vi "2.4.vi"() -> ()   [LabVIEW 2020]
panel:
  out "DIVISION":string
  out "PRODUCTO  2":string
  out "RESTA":string
  out "SUMA":string
  in  "Numero B":dbl
  in  "Numero A":dbl
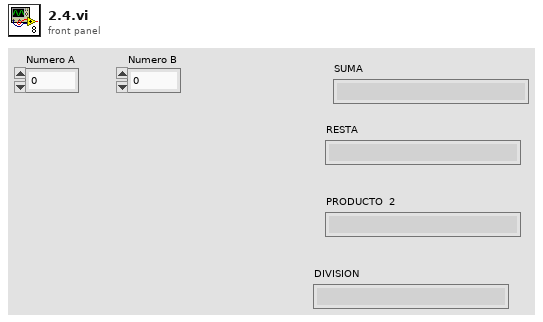
[diagram p1: front panel]
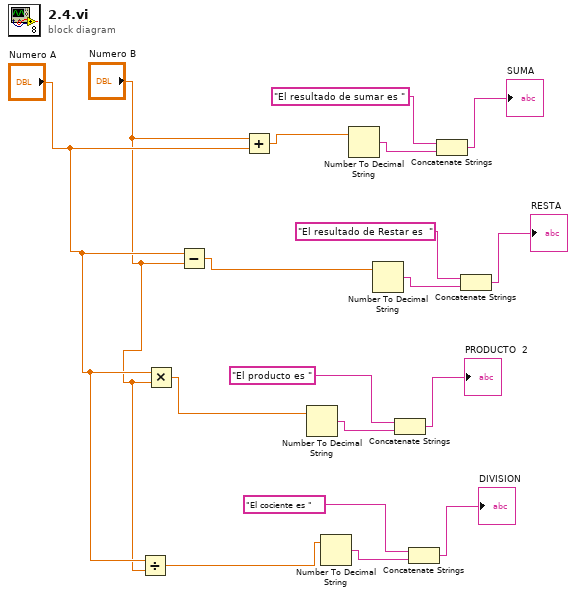
[diagram p0: block diagram]
diagram:
  n1 = Divide(x="Numero A", y="Numero B") -> (x/y=w1:dbl)
  n2 = Multiply(x="Numero A", y="Numero B") -> (x*y=w2:dbl)
  n3 = Subtract(x="Numero A", y="Numero B") -> (x-y=w5:dbl)
  n4 = Add(x="Numero B", y="Numero A") -> (x+y=w18:dbl)
  n5 = Number To Decimal String(number=w2) -> (decimal integer string=w9:string)  [unwired: 1 in]
  n6 = Number To Decimal String(number=w1) -> (decimal integer string=w6:string)  [unwired: 1 in]
  n7 = Number To Decimal String(number=w18) -> (decimal integer string=w15:string)  [unwired: 1 in]
  n8 = Number To Decimal String(number=w5) -> (decimal integer string=w12:string)  [unwired: 1 in]
  n9 = Concatenate Strings("El producto es ", w9) -> (→"PRODUCTO  2":string)
  n10 = Concatenate Strings("El cociente es ", w6) -> (→"DIVISION":string)
  n11 = Concatenate Strings("El resultado de sumar es ", w15) -> (→"SUMA":string)
  n12 = Concatenate Strings("El resultado de Restar es  ", w12) -> (→"RESTA":string)
